vi "empty.vi"(11 "Array":dbl[](array[numeric])) -> (3 "output":dbl[](array[numeric]))   [LabVIEW 2013]
panel:
  in  "empty_array":dbl[](array[numeric])
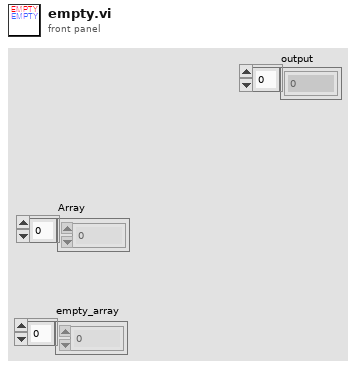
[diagram p1: front panel]
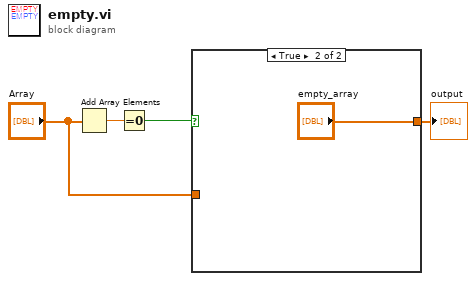
[diagram p0: block diagram]
diagram:
  n1 = Add Array Elements(numeric array="Array") -> (sum=w4:dbl)
  n2 = Equal To 0?(x=w4) -> (x = 0?=w3:bool)
  n3 = case shown="True" w3 {
    tunnel: "Array" -> [w5 _]
    tunnel: [w5 "empty_array"] -> w1
    frame False {
    }
    frame True {
    }
  }
  "output" <- w1
